vi "Shutdown.vi"(8 "error in (no error)":errorcluster, 11 "VolatusAPI in":refnum<class "VolatusAPI.lvclass">) -> (0 "error out":errorcluster, 3 "VolatusAPI out":refnum<class "VolatusAPI.lvclass">)   [LabVIEW 2020, in "Volatus.lvlib" / "VolatusAPI.lvclass"]
uses:
  VolatusAPI.lvclass
  Volatus Core Identity/Volatus Core Identity.lvclass
  C:/dev/lv20CE/relink/lv-volatus/Volatus/Identity/Identity.lvclass
  Volatus.lvlib
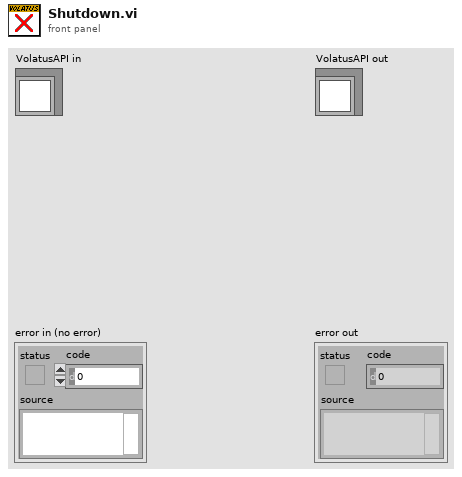
[diagram p1: front panel]
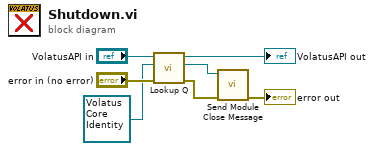
[diagram p0: block diagram]
diagram:
  n1 = call "Lookup Q.vi"("error in (no error)"="error in (no error)", "Identity"=refnum<class "Volatus Core Identity.lvclass"> refnum ("Volatus:Volatus Core Identity.lvclass"), "VolatusAPI in"="VolatusAPI in") -> ("error out"=w2:errorcluster, "MessageQ"=w3:refnum<class "MessageQ.lvclass">, "VolatusAPI out"=→"VolatusAPI out":refnum<class "VolatusAPI.lvclass">)  [unwired: 6 in]
  n2 = call "Send Module Close Message.vi"("error in (no error)"=w2, "MessageQ"=w3) -> ("error out"=→"error out":errorcluster)  [unwired: 9 in]
